vi "Get Power Meter Default Value.vi"(0 "SG Path PM Accessor in":refnum<class "SG Path Accessor.lvclass">, 11 "error in":errorcluster) -> (4 "SG Path PM Accessor out":refnum<class "SG Path Accessor.lvclass">, 6 "Power Meter out":refnum<class "Power Meter Base.lvclass">, 15 "error out":errorcluster)   [LabVIEW 2023, in "RS NRPx Power Meter.lvlib" / "SG Path Accessor.lvclass"]
uses:
  SG Path Accessor.lvclass
  Instruments/Power Meter/Power Meter Base/Power Meter Base.lvclass
  Power Meter/Power Meter.lvclass
  C:/srd-semi-rfcal-software/AuxTools/STSRFFixtureCharactUtility/Source/Code Modules/Fixture/Instruments/Power Meter/Power Meter Base/Power Meter Base.lvclass
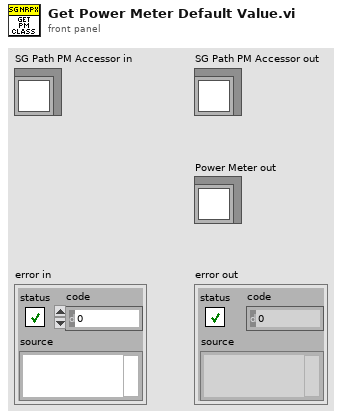
[diagram p1: front panel]
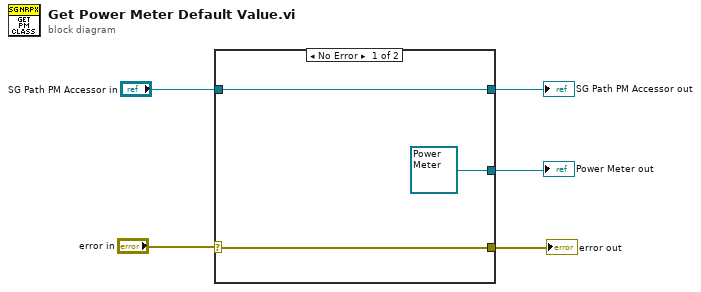
[diagram p0: block diagram]
diagram:
  n1 = case shown="No Error" "error in" {
    selector: "error in" -> [w6 w9]
    tunnel: "SG Path PM Accessor in" -> [w7 w10]
    tunnel: [w7 w10] -> w3
    tunnel: [w6 w9] -> w1
    tunnel: [refnum<class "Power Meter.lvclass"> refnum ("STS Scalar Fixture Charact.lvlib:PM NI568X.lvclass") _] -> w2
    frame No Error {
    }
    frame Error {
    }
  }
  "error out" <- w1
  "SG Path PM Accessor out" <- w3
  "Power Meter out" <- w2
